vi "Read SCH Secondary Parameters MGI RWA.vi"(8 "error in (no error)":errorcluster, 10 "Done":bool, 11 "FPGA Refnum in":T2) -> (0 "error out":errorcluster, 3 "Refnum out":T2)   [LabVIEW 2018]
doc: "Author: Scott Hannahs <sth@magnet.fsu.edu>\nCopyright 2018 Florida State University, All rights reserved."
uses:
  RT Controls/FPGA SCH Secondary Digitizer Ref.ctl
  SCH Data Controls/FPGA Secondary Configure Parameters.ctl
  <userlib>/_MGI/Read Write Anything/MGI RWA Options Cluster.ctl
panel:
  in  "FPGA Secondary Configuration Values":T1={"Ln2 Filter Size"=10, "CoWound Volt Limit"=0.2000122070312, "CoWound Tick Limit"=4000000, "DAQ Cycle Ticks"=4096, "Co-Wound Asymmetry Factor"=-0.0026654, "Co-Wound Scale Factor"=59.952, "# Consecutive Zeros Fault"=1000, "Digitize Convert Ticks"=200, "Digitize Reset Ticks"=400, "Convert Clock Ticks"=20, "Digitize Read Delay Ticks"=41, "Digitize # Bits"=16, "Low Current (kA)"=0.04500000178814, "Low Current Ticks"=400000000, "Low Current Delay Factor"=100, "Cold Mass Scale Factor"=59.988, "Current Scale Factor"=2.0} {"Current Scale Factor" format="%_6g"; "Co-Wound Asymmetry Factor" format="%.8g"}
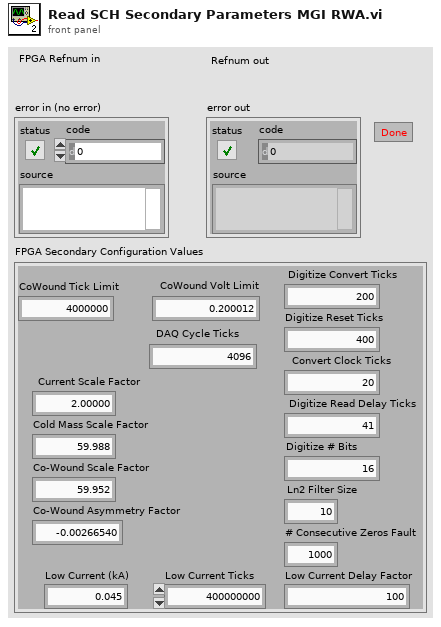
[diagram p1: front panel]
types:
  T1 = typedef "FPGA Secondary Configure Parameters.ctl" = cluster{"Ln2 Filter Size":i16, "CoWound Volt Limit":dbl, "CoWound Tick Limit":u32, "DAQ Cycle Ticks":u32, "Co-Wound Asymmetry Factor":dbl, "Co-Wound Scale Factor":dbl, "# Consecutive Zeros Fault":i16, "Digitize Convert Ticks":u32, "Digitize Reset Ticks":u32, "Convert Clock Ticks":u32, "Digitize Read Delay Ticks":u32, "Digitize # Bits":u32, "Low Current (kA)":dbl, "Low Current Ticks":u32, "Low Current Delay Factor":u16, "Cold Mass Scale Factor":dbl, "Current Scale Factor":dbl}
  T2 = typedef "FPGA SCH Secondary Digitizer Ref.ctl" = refnum<k20>
  T3 = typedef "MGI RWA Options Cluster.ctl" = cluster{"TS Fmt":string, "Int Fmt":string, "Delimiter":string}
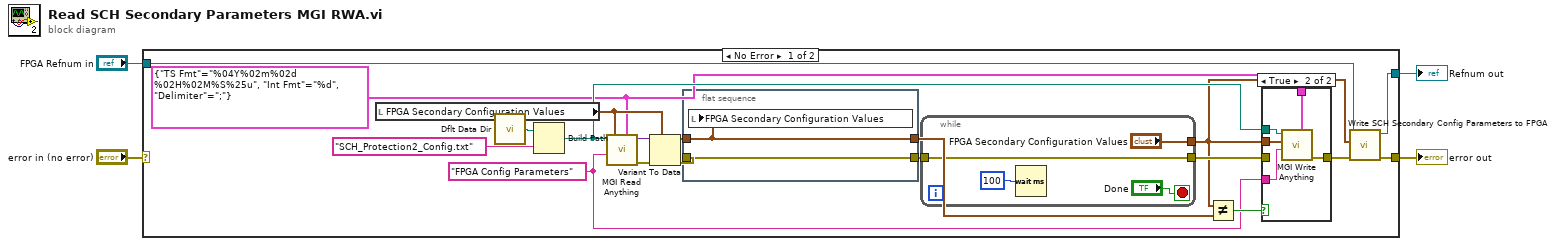
[diagram p0: block diagram]
diagram:
  n1 = case shown="No Error" "error in (no error)" {
    selector: "error in (no error)" -> [_ w37]
    tunnel: [w10 w37] -> w3
    tunnel: "FPGA Refnum in" -> [w5 w36]
    tunnel: [w8 w36] -> w1
    frame No Error {
      w6 = T3 {"TS Fmt"="%04Y%02m%02d %02H%02M%S%25u", "Int Fmt"="%d", "Delimiter"=";"} ("Read/Write Options (Version 1.x)")
      w13 = "FPGA Config Parameters" ("section")
      n2 = local read "FPGA Secondary Configuration Values"() -> (w16:T1)
      n3 = call <vilib>:"Dflt Data Dir.vi"() -> ("App:Default Data Directory"=w23:path)
      n4 = Build Path(base path=w23, name or relative path="SCH_Protection2_Config.txt") -> (appended path=w12:path)
      n5 = call <userlib>:"MGI Read Anything.vi"("Read/Write Options (Version 1.x)"=w6, "Type of Anything"=w16, "Section Name (Name of \"Type of Anything\")"=w13, "Path (dialog)"=w12) -> ("Error Out"=w7:errorcluster, "Anything"=w17:variant)  [unwired: 4 in, 2 out]
      n6 = Variant To Data(error in=w7, type=w16, Variant=w17) -> (data=w15:T1, error out=w14:errorcluster)
      n7 = flat-sequence {
        tunnel: [w24] -> w21
        tunnel: [w25] -> w20
        tunnel: w15 -> [w25]
        tunnel: w14 -> [w24]
        frame #0 {
          n8 = local write "FPGA Secondary Configuration Values"(w25) -> ()
        }
      }
      n9 = while {
        tunnel: w21 -> [w35]
        tunnel: [w35] -> w18
        tunnel: ["FPGA Secondary Configuration Values"] -> w9
        stop <- "Done" stop-if-true
        n10 = Wait (ms)(milliseconds to wait=u32 100) -> ()  [unwired: 1 out]
      }
      n11 = Not Equal?(x=w9, y=w20) -> (x != y?=w19:bool)
      n12 = case shown="True" w19 {
        tunnel: w18 -> [w26 _]
        tunnel: w9 -> [_ w28]
        tunnel: [w26 w29] -> w11
        tunnel: w13 -> [_ w31]
        tunnel: w12 -> [_ w30]
        tunnel: w6 -> [_ w27]
        frame False {
        }
        frame True {
          n13 = call <userlib>:"MGI Write Anything.vi"("Read/Write Options"=w27, "Section Name (Name of \"Anything\")"=w31, "Anything"=w28, "Path (dialog)"=w30) -> ("Error Out"=w29:errorcluster)  [unwired: 5 in, 2 out]
        }
      }
      n14 = call "Write SCH Secondary Config Parameters to FPGA.vi"("error in (no error)"=w11, "FPGA Configuration Values"=w9, "Refnum in"=w5) -> ("error out"=w10:errorcluster, "Refnum out"=w8:T2)  [unwired: 7 in]
    }
    frame Error {
    }
  }
  "Refnum out" <- w1
  "error out" <- w3
